vi "start calculate.vi"(8 "lenght":dbl[](array[numeric]), 9 "start":dbl[](array[numeric]), 11 "act":bool[](array[boolean])) -> (0 "最大值":i32, 2 "width":i32[](array[numeric]), 3 "begin":i32[](array[numeric]))   [LabVIEW 2018]
panel:
  out "数组 3":i32[](array[numeric])
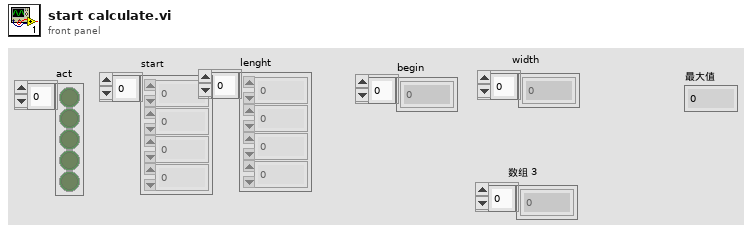
[diagram p1: front panel]
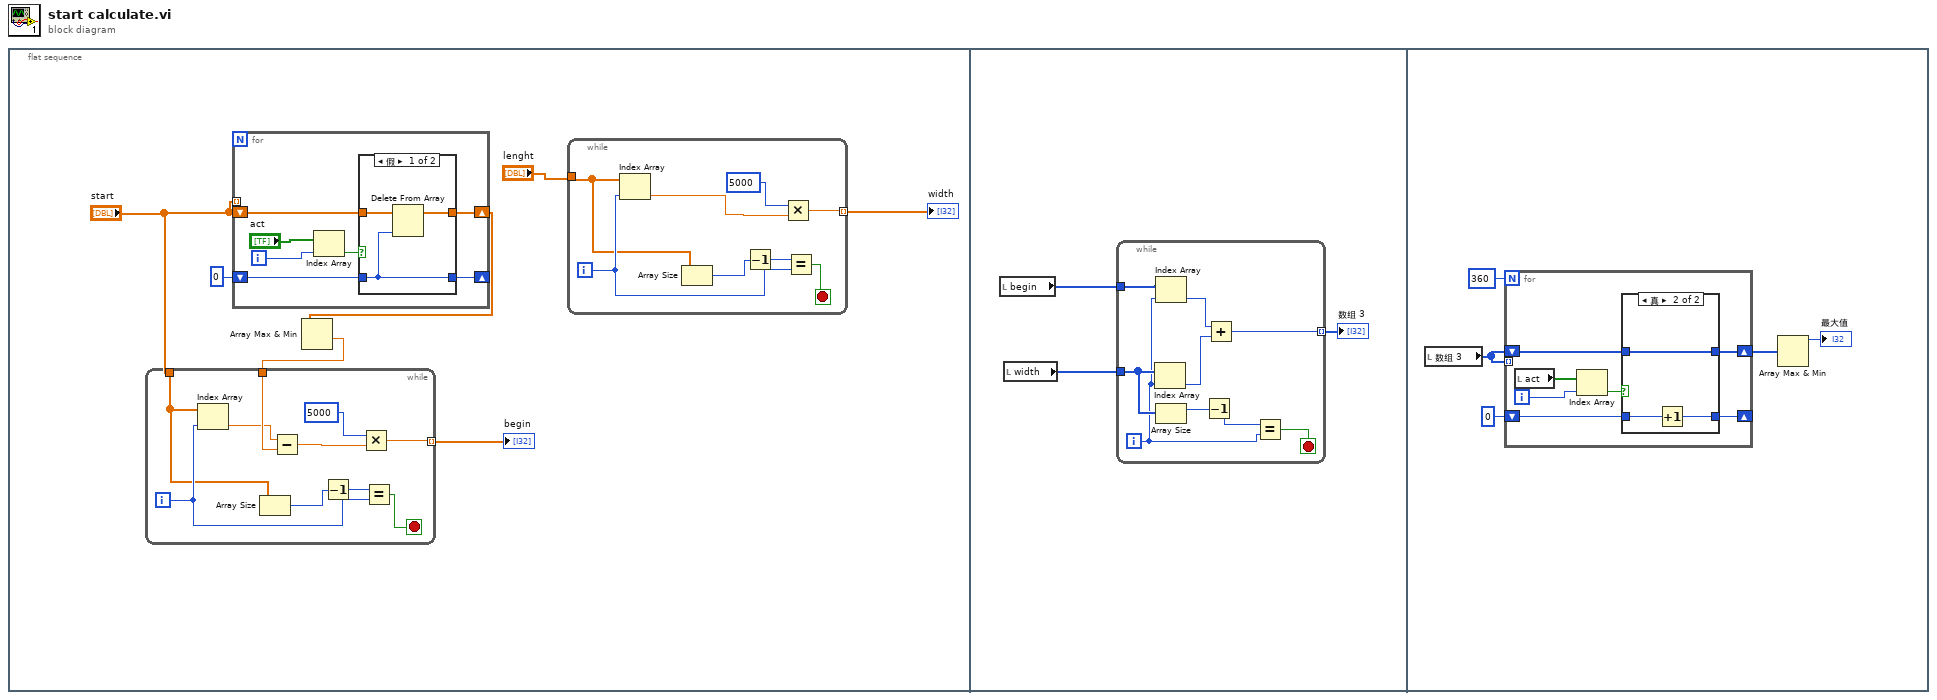
[diagram p0: block diagram]
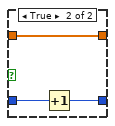
[diagram p2: hidden frame]
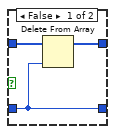
[diagram p3: hidden frame]
diagram:
  n1 = flat-sequence {
    frame #0 {
      n2 = for {
        shift-right: [w30] -> w6
        shift-left: "start" -> [w31]
        tunnel: "start" -> [_] mode=indexing
        shift-right: [w27] -> _
        shift-left: u8 0 -> [w28]
        i -> [w29]
        n3 = Index Array(array="act", index=w29) -> (element=w32:bool)
        n4 = case shown="假" w32 {
          tunnel: w31 -> [w35 w38]
          tunnel: [w34 w38] -> w30
          tunnel: w28 -> [w33 w37]
          tunnel: [w33 w36] -> w27
          frame False {
            n5 = Delete From Array(array=w35, index=w33) -> (array with subset deleted=w34:dbl[])  [unwired: 1 in, 1 out]
          }
          frame True {
            n6 = Increment(x=w37) -> (x+1=w36:u8)
          }
        }
      }
      n7 = Array Max & Min(array=w6) -> (min value=w5:dbl)  [unwired: 3 out]
      n8 = while {
        tunnel: "start" -> [w18]
        tunnel: w5 -> [w25]
        tunnel: [w16] -> w4 mode=indexing
        i -> [w19]
        stop <- w17 stop-if-true
        n9 = Index Array(array=w18, index=w19) -> (element=w24:dbl)
        n10 = Array Size(array=w18) -> (size(s)=w20:i32)
        n11 = Subtract(x=w24, y=w25) -> (x-y=w23:dbl)
        n12 = Decrement(x=w20) -> (x-1=w21:i32)
        n13 = Multiply(x=5000, y=w23) -> (x*y=w16:dbl)
        n14 = Equal?(x=w21, y=w19) -> (x = y?=w17:bool)
      }
      "begin" <- w4
      n15 = while {
        tunnel: "lenght" -> [w11]
        tunnel: [w9] -> w3 mode=indexing
        i -> [w12]
        stop <- w10 stop-if-true
        n16 = Index Array(array=w11, index=w12) -> (element=w8:dbl)
        n17 = Array Size(array=w11) -> (size(s)=w13:i32)
        n18 = Decrement(x=w13) -> (x-1=w14:i32)
        n19 = Multiply(x=5000, y=w8) -> (x*y=w9:dbl)
        n20 = Equal?(x=w14, y=w12) -> (x = y?=w10:bool)
      }
      "width" <- w3
    }
    frame #1 {
      n21 = local read "begin"() -> (w39:i32[])
      n22 = local read "width"() -> (w40:i32[])
      n23 = while {
        tunnel: w39 -> [w50]
        tunnel: w40 -> [w49]
        tunnel: [w42] -> w41 mode=indexing
        i -> [w46]
        stop <- w45 stop-if-true
        n24 = Index Array(array=w49, index=w46) -> (element=w43:i32)
        n25 = Index Array(array=w50, index=w46) -> (element=w44:i32)
        n26 = Array Size(array=w49) -> (size(s)=w47:i32)
        n27 = Decrement(x=w47) -> (x-1=w48:i32)
        n28 = Add(x=w44, y=w43) -> (x+y=w42:i32)
        n29 = Equal?(x=w48, y=w46) -> (x = y?=w45:bool)
      }
      "数组 3" <- w41
    }
    frame #2 {
      n30 = local read "数组 3"() -> (w53:i32[])
      n31 = for {
        N: 360 -> [_]
        shift-right: [w59] -> w54
        shift-left: w53 -> [w60]
        shift-right: [w56] -> _
        shift-left: u8 0 -> [w57]
        tunnel: w53 -> [_] mode=indexing
        i -> [w58]
        n32 = local read "act"() -> (w62:bool[])
        n33 = Index Array(array=w62, index=w58) -> (element=w61:bool)
        n34 = case shown="真" w61 {
          tunnel: w60 -> [w65 w68]
          tunnel: [w64 w68] -> w59
          tunnel: w57 -> [w63 w67]
          tunnel: [w63 w66] -> w56
          frame False {
            n35 = Delete From Array(array=w65, index=w63) -> (array with subset deleted=w64:i32[])  [unwired: 1 in, 1 out]
          }
          frame True {
            n36 = Increment(x=w67) -> (x+1=w66:u8)
          }
        }
      }
      n37 = Array Max & Min(array=w54) -> (max value=→"最大值":i32)  [unwired: 3 out]
    }
  }
